vi "Finish Trace.vi"(5 "Values":refnum<class "Values.lvclass">, 7 "Response":refnum<class "Response.lvclass">, 8 "error in (no error)":errorcluster, 10 "Session Debug Info":T1, 11 "RequestTraceLog in":refnum<class "RequestTraceLog.lvclass">) -> (0 "error out":errorcluster, 3 "RequestTraceLog out":refnum<class "RequestTraceLog.lvclass">)   [LabVIEW 2020, in "HTTP Server.lvlib" / "RequestTraceLog.lvclass"]
uses:
  RequestTraceLog.lvclass
  <vilib>/IlluminatedG/IG HTTP Utils/HTTP Utils/Response/Response.lvclass
  Values/Values.lvclass
  Session Debug Info.ctl
  Security/Security.lvclass
  C:/dev/lv/2020/lv-http-server/HTTP Server/Service/Service.lvclass
  User/User.lvclass
  RequestTraceLog.lvclass/RequestTraceLog.ctl
  HTTP Server.lvlib
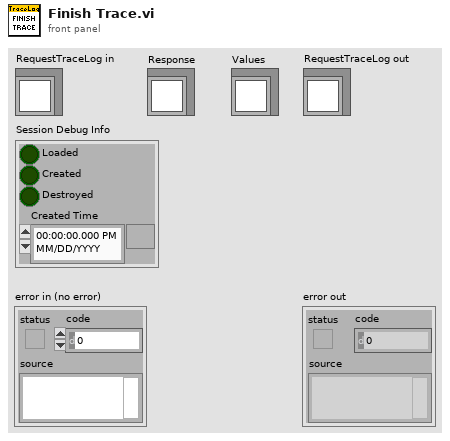
[diagram p1: front panel]
types:
  T1 = typedef "HTTP Server.lvlib/Session Debug Info.ctl" = cluster{"Loaded":bool, "Created":bool, "Destroyed":bool, "Created Time":timestamp}
  T2 = typedef "HTTP Server.lvlib/Trace Item.ctl" = cluster{"Duration":dbl, "Step":T3, "Class":string, "Info":string, "Status":bool, "Code":i32, "Time":dbl}
  T3 = typedef "HTTP Server.lvlib/Processing Step.ctl" = enum16{"Connection", "Request", "Routing", "Controller Init", "Controller", "Response", "Complete", "Exception"}
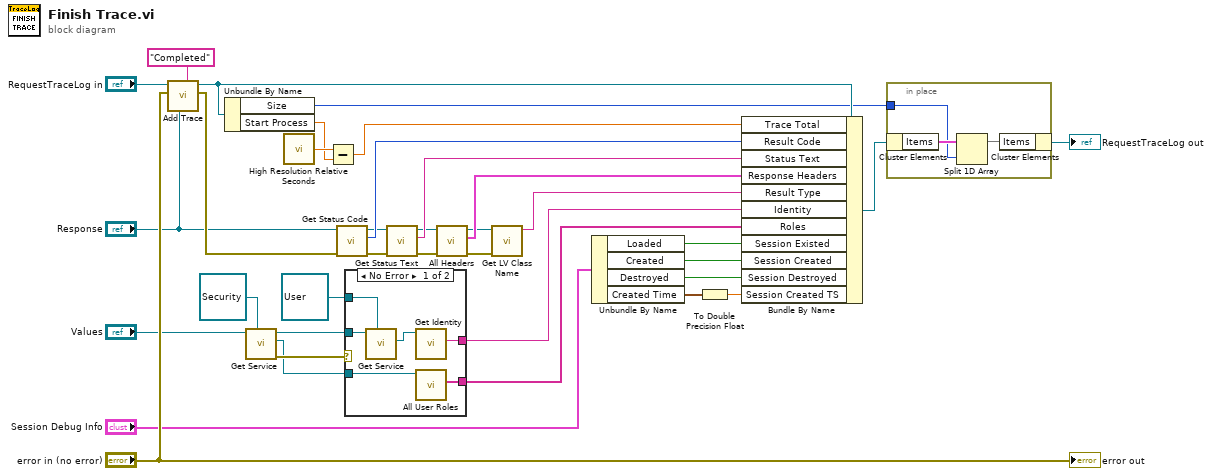
[diagram p0: block diagram]
diagram:
  n1 = call "Add Trace.vi"("Info"="Completed", "LabVIEW Object"="Response", "error in (no error)"="error in (no error)", "RequestTraceLog in"="RequestTraceLog in") -> ("error out"=w36:errorcluster, "RequestTraceLog out"=w28:refnum<class "RequestTraceLog.lvclass">)  [unwired: 6 in]
  n2 = Unbundle By Name(w28) -> ("Size"=w27:i32, "Start Process"=w24:dbl)
  n3 = call "Get Service.vi"("Service Type"=refnum<class "Security.lvclass"> refnum ("HTTP Server.lvlib:Security.lvclass"), "Values in"="Values") -> ("error out"=w12:errorcluster, "Service"=w10:refnum<class "Security.lvclass">, "Values out"=w11:refnum<class "Values.lvclass">)  [unwired: 7 in]
  n4 = call <vilib>:"High Resolution Relative Seconds.vi"() -> ("relative seconds"=w25:dbl)
  n5 = Subtract(x=w25, y=w24) -> (x-y=w23:dbl)
  n6 = call <vilib>:"Get Status Code.vi"("error in (no error)"=w36, "Response in"="Response") -> ("error out"=w20:errorcluster, "Status Code"=w33:u16, "Response out"=w22:refnum<class "Response.lvclass">)  [unwired: 7 in]
  n7 = case shown="No Error" w12 {
    tunnel: w11 -> [w42 _]
    tunnel: w10 -> [w41 _]
    tunnel: [w39 _] -> w9
    tunnel: [w38 _] -> w7
    tunnel: refnum<class "User.lvclass"> refnum ("HTTP Server.lvlib:User.lvclass") -> [w37 _]
    frame No Error {
      n8 = call "Get Service.vi"("Service Type"=w37, "Values in"=w42) -> ("Service"=w40:refnum<class "User.lvclass">)  [unwired: 7 in, 2 out]
      n9 = call-dynamic "Get Identity.vi"("User in"=w40) -> ("Identity"=w39:string)  [unwired: 8 in, 2 out]
      n10 = call "All User Roles.vi"("Security in"=w41) -> ("User Roles"=w38:string[])  [unwired: 8 in, 2 out]
    }
    frame Error {
    }
  }
  n11 = call <vilib>:"Get Status Text.vi"("error in (no error)"=w20, "Response in"=w22) -> ("error out"=w18:errorcluster, "Status Text"=w21:string, "Response out"=w19:refnum<class "Response.lvclass">)  [unwired: 7 in]
  n12 = call <vilib>:"All Headers.vi"("error in (no error)"=w18, "Response in"=w19) -> ("error out"=w15:errorcluster, "Headers"=w17:cluster{"Header":string, "Value":string}[], "Response out"=w16:refnum<class "Response.lvclass">)  [unwired: 7 in]
  n13 = call <vilib>:"Get LV Class Name.vi"("error in (no error)"=w15, "object"=w16) -> ("class name"=w34:string)  [unwired: 8 in, 1 out]
  n14 = Unbundle By Name("Session Debug Info") -> ("Loaded"=w4:bool, "Created"=w3:bool, "Destroyed"=w2:bool, "Created Time"=w1:timestamp)
  n15 = To Double Precision Float(number=w1) -> (double precision float=w6:dbl)
  n16 = Bundle By Name(cluster=w28, "Trace Total"=w23, "Result Code"=w33, "Status Text"=w21, "Response Headers"=w17, "Result Type"=w34, "Identity"=w9, "Roles"=w7, "Session Existed"=w4, "Session Created"=w3, "Session Destroyed"=w2, "Session Created TS"=w6) -> (w32:refnum<class "RequestTraceLog.lvclass">)
  n17 = in-place {
    in-place-border: w27 -> [w44]
    n18 = in-place-cluster #1(w32) -> ("Items"=w45:T2[])
    n19 = Split 1D Array(array=w45, index=w44) -> (first subarray=w43:T2[])  [unwired: 1 out]
    n20 = in-place-cluster #1("Items"=w43) -> (→"RequestTraceLog out":refnum<class "RequestTraceLog.lvclass">)
  }
  "error out" <- "error in (no error)"
